vi "Place_Element_In_1D_Array_Str.vi"(1 "element":string, 2 "index":i32, 3 "String array in":string[](array[string])) -> (0 "String output array":string[](array[string]))   [LabVIEW 2011, in "Third Party VIs.lvlib" / "pcardinale.lvlib"]
doc: "Places an element in a 1-D array, either by replacing and existing element. or padding and appending."
uses:
  pcardinale.lvlib
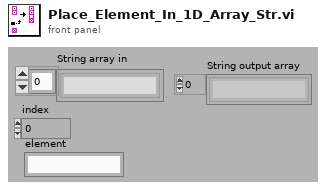
[diagram p1: front panel]
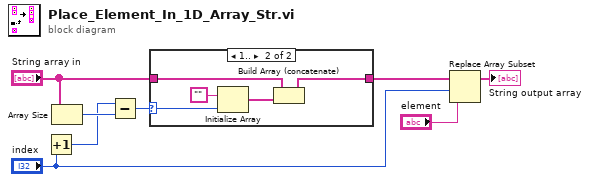
[diagram p0: block diagram]
diagram:
  n1 = Increment(x="index") -> (x+1=w6:i32)
  n2 = Array Size(array="String array in") -> (size(s)=w7:i32)
  n3 = Subtract(x=w6, y=w7) -> (x-y=w5:i32)
  n4 = case shown="1.." w5 {
    selector: w5 -> [_ w14]
    tunnel: "String array in" -> [w9 w13]
    tunnel: [w9 w11] -> w4
    frame ..0, Default {
    }
    frame 1.. {
      n5 = Initialize Array("", w14) -> (w12:string[])
      n6 = Build Array (concatenate)(w13, w12) -> (w11:string[])
    }
  }
  n7 = Replace Array Subset(array=w4, new element="element", index="index") -> (→"String output array":string[])
